vi "Main.vi"(11 "Module Admin":refnum<class "Delacor_lib_QMH_Cloneable Module Admin.lvclass">) -> ()   [LabVIEW 2025, in "Wheatstone Bridge.lvlib"]
doc: "This template is based off of the Queued Message Handler design pattern and the Queued Message Handler project template that ships with LabVIEW.\n\nThe main difference is that the queue is private to this module and communication between modules is performed via Broadcast and Request events.\n\nRequest events are wrapped in public API methods and are handled in the Event Handling Loop (EHL) of this VI. Any module can register for Broadcast events sent by this module. The EHL generates messages based on user interface actions.\n\nThe Message Handling Loop (MHL) processes messages generated by the EHL, or by other messages. The messages are string values, so new messages can be added easily to the Message Cases case structure in the MHL. Each message cluster can also provide an optional value for Message Data, which is a variant that can be converted to whatever message-specific data is required.\n_____\nBased on DQMH Dev Tools: Project Template 7.1.2.1547."
uses:
  Wheatstone Bridge.lvlib
  <vilib>/Delacor/Delacor QMH/Libraries/Message Queue_class/Delacor_lib_QMH_Message Queue.lvclass
  Module Data--cluster.ctl
  <vilib>/Utility/miscctls.llb/LVPointTypeDef.ctl
  <vilib>/Delacor/Delacor QMH/Libraries/Message Queue_class/Delacor_lib_QMH_Enqueue Message (Single).vi
  Stop Argument--cluster.ctl
  <vilib>/Delacor/Delacor QMH/Libraries/Cloneable Module Admin_class/Delacor_lib_QMH_Cloneable Module Admin.lvclass
  select child (Reply Payload)--cluster.ctl
  Wheatstone Bridge/Hardware Selection.ctl
  Wheatstone Bridge/Wheatstone Bridge.lvclass
  select child Argument--cluster.ctl
  NI-9237/NI-9237.lvclass
  read config (Reply Payload)--cluster.ctl
  read config Argument--cluster.ctl
  init device (Reply Payload)--cluster.ctl
  init device Argument--cluster.ctl
  close (Reply Payload)--cluster.ctl
  close Argument--cluster.ctl
  read data (Reply Payload)--cluster.ctl
  read data Argument--cluster.ctl
  read dvr (Reply Payload)--cluster.ctl
  read dvr Argument--cluster.ctl
  C:/Users/Tyson.Grover/Desktop/Repositories/torque-test-station/Libraries/Wheatstone Bridge/Wheatstone Bridge/Wheatstone Bridge.lvclass
  C:/Users/Tyson.Grover/Desktop/Repositories/torque-test-station/Libraries/Wheatstone Bridge/NI-9237/NI-9237.lvclass
panel:
  out "Stop the VI":bool
  out "Data Cluster":T1={"Status"="Inactive", "Wheatstone Bridge"=refnum}
  out "error out":errorcluster
  out "Status":string
  in  "Simulate EHL Error":bool
  in  "Simulate MHL Error":bool
  # "Other processes communicate with this Module via its Public API (wrappers for its Request Events).\n\nThis Module communicates with other processes via its Broadcast Events.\nAny process that wants to receive these messages can register for this module's Broadcast events."
  # "This template is for the DQMH framework. See the block diagram for more information on how to use this template."
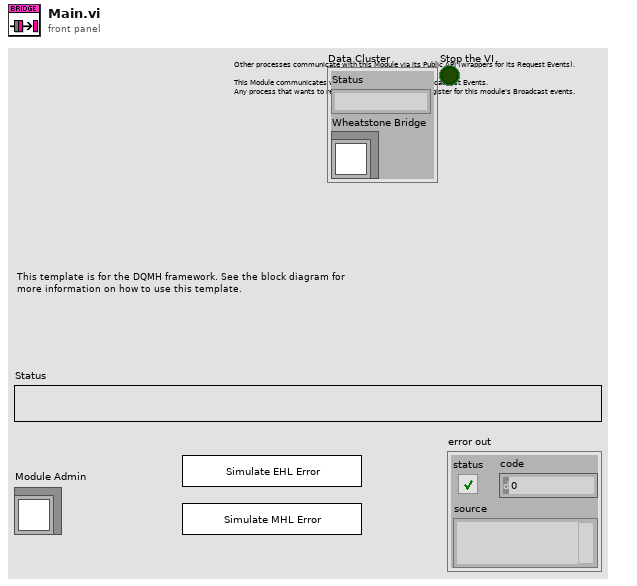
[diagram p1: front panel]
types:
  T1 = typedef "Wheatstone Bridge.lvlib/Module Data--cluster.ctl" = cluster{"Status":string, "Wheatstone Bridge":refnum<class "Wheatstone Bridge.lvclass">}
  T2 = typedef "Wheatstone Bridge.lvlib/Request Events--cluster.ctl" = cluster{"Stop Module":refnum<user-event>, "Show Panel":refnum<user-event>, "Hide Panel":refnum<user-event>, "Show Diagram":refnum<user-event>, "Get Module Execution Status":refnum<user-event>, "select child":refnum<user-event>, "read config":refnum<user-event>, "init":refnum<user-event>, "init device":refnum<user-event>, "close":refnum<user-event>, "read data":refnum<user-event>, "read dvr":refnum<user-event>}
  T3 = enum32{"invalid lock state", "Not Locked", "Locked (No Password)", "Password-protected"}
  T4 = typedef "Wheatstone Bridge.lvlib/Stop Argument--cluster.ctl" = cluster{"Module ID":i32, "Origin":string, "Exit via Stop Module Req?":bool, "Wait for Module to stop?":bool}
  T5 = typedef "Wheatstone Bridge.lvlib/select child Argument--cluster.ctl" = cluster{"Module ID":i32, "Hardware Selection":T6, "Wait Notifier":refnum<notifier>, "wait for reply":bool}
  T6 = typedef "Wheatstone Bridge.lvlib/Wheatstone Bridge.lvclass/Hardware Selection.ctl" = enum16{"Wheatstone Bridge", "NI-9237"}
  T7 = typedef "Wheatstone Bridge.lvlib/read config Argument--cluster.ctl" = cluster{"Module ID":i32, "File Path":path, "Wait Notifier":refnum<notifier>, "wait for reply":bool}
  T8 = typedef "Wheatstone Bridge.lvlib/init device Argument--cluster.ctl" = cluster{"Module ID":i32, "Variant":variant, "Wait Notifier":refnum<notifier>, "wait for reply":bool}
  T9 = typedef "Wheatstone Bridge.lvlib/close Argument--cluster.ctl" = cluster{"Module ID":i32, "Wait Notifier":refnum<notifier>, "wait for reply":bool}
  T10 = typedef "Wheatstone Bridge.lvlib/read data Argument--cluster.ctl" = cluster{"Module ID":i32, "Wait Notifier":refnum<notifier>, "wait for reply":bool}
  T11 = typedef "Wheatstone Bridge.lvlib/read dvr Argument--cluster.ctl" = cluster{"Module ID":i32, "Wait Notifier":refnum<notifier>, "wait for reply":bool}
  T12 = typedef "LVPointTypeDef.ctl" = cluster{"Horizontal":i16, "Vertical":i16}
  T13 = enum32{"Invalid", "Standard", "Closed", "Hidden", "Minimized", "Maximized"}
  T14 = typedef "Wheatstone Bridge.lvlib/select child (Reply Payload)--cluster.ctl" = cluster{"Module ID":i32, "error":errorcluster}
  T15 = typedef "Wheatstone Bridge.lvlib/read config (Reply Payload)--cluster.ctl" = cluster{"Module ID":i32, "error":errorcluster}
  T16 = typedef "Wheatstone Bridge.lvlib/init device (Reply Payload)--cluster.ctl" = cluster{"Module ID":i32, "error":errorcluster}
  T17 = typedef "Wheatstone Bridge.lvlib/close (Reply Payload)--cluster.ctl" = cluster{"Module ID":i32, "error":errorcluster}
  T18 = typedef "Wheatstone Bridge.lvlib/read data (Reply Payload)--cluster.ctl" = cluster{"Module ID":i32, "error":errorcluster}
  T19 = typedef "Wheatstone Bridge.lvlib/read dvr (Reply Payload)--cluster.ctl" = cluster{"Module ID":i32, "Numeric":dbl, "error":errorcluster}
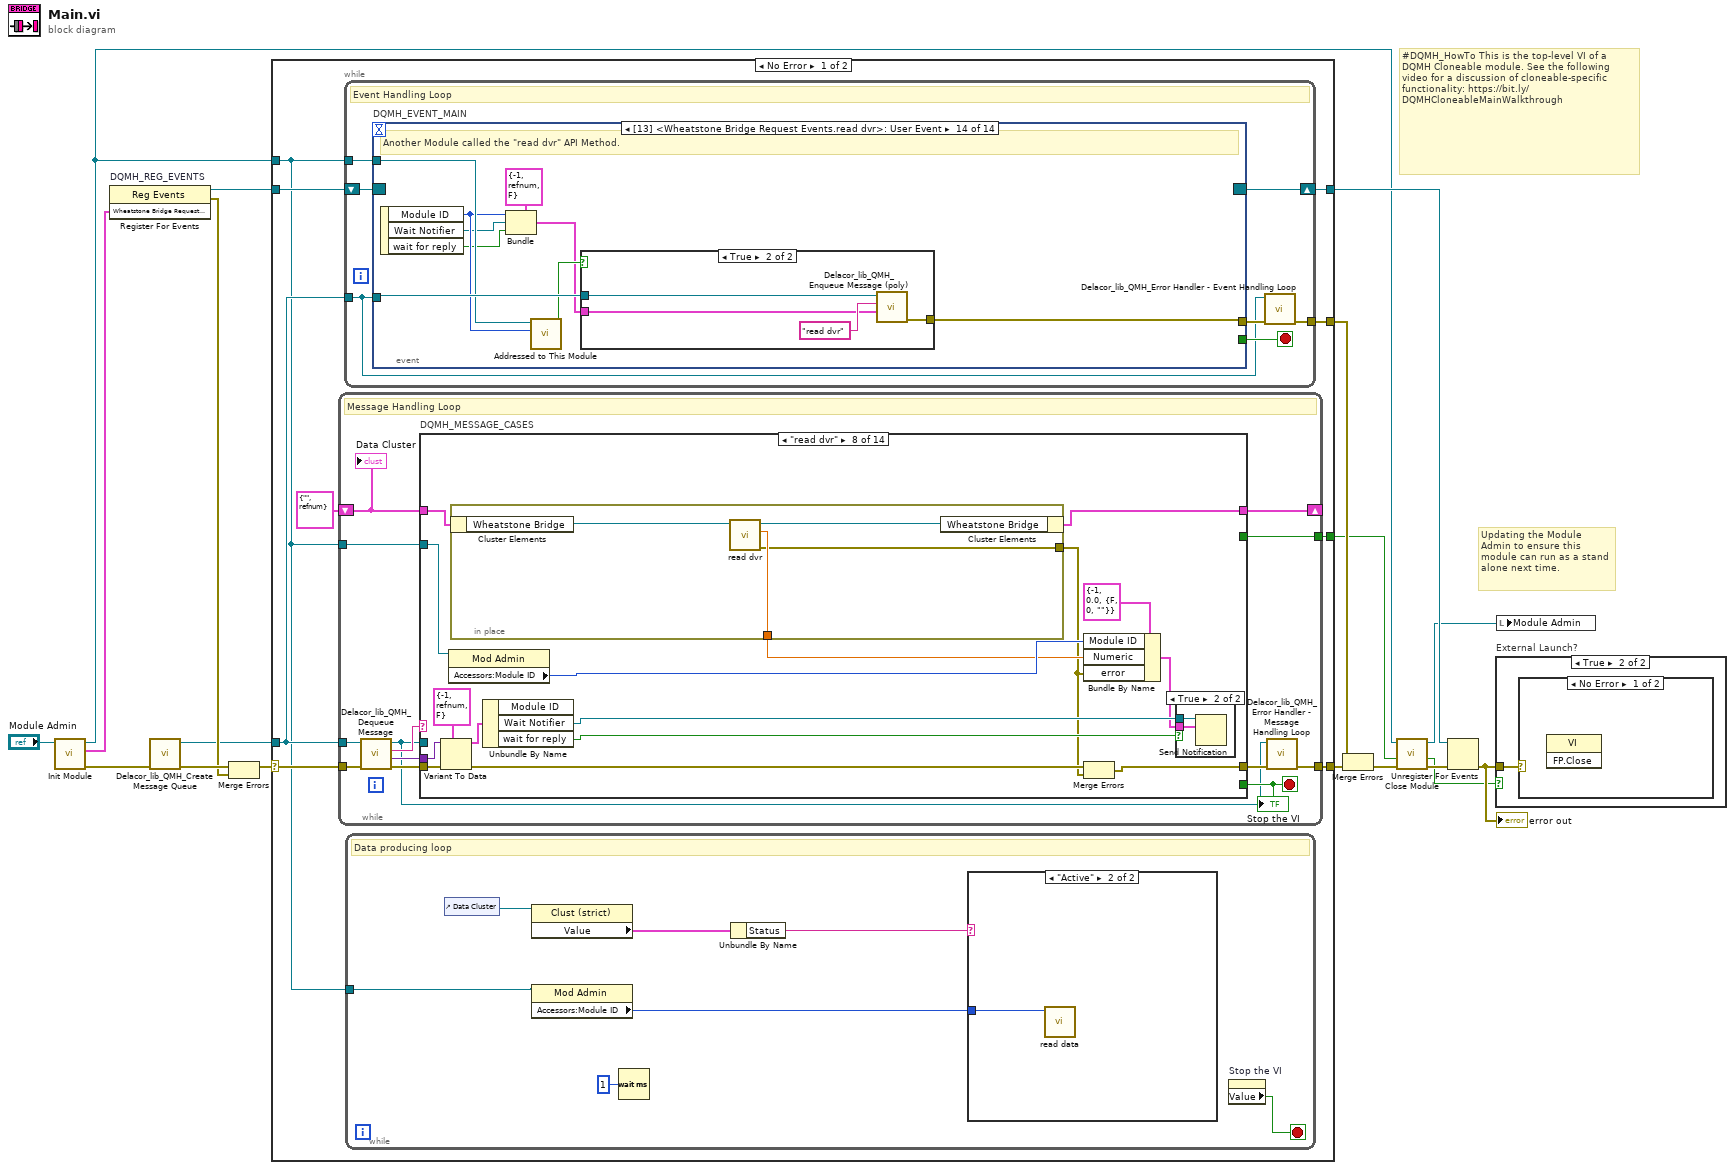
[diagram p0: block diagram]
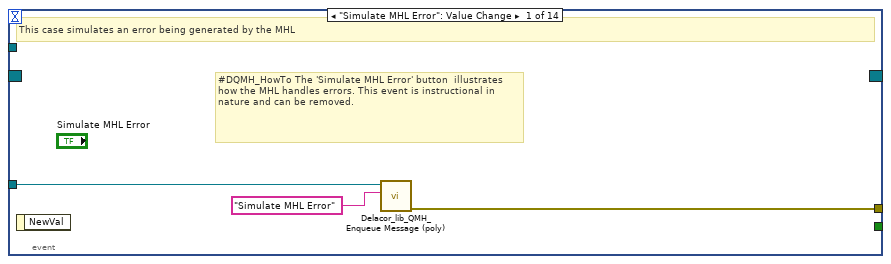
[diagram p3: hidden frame]
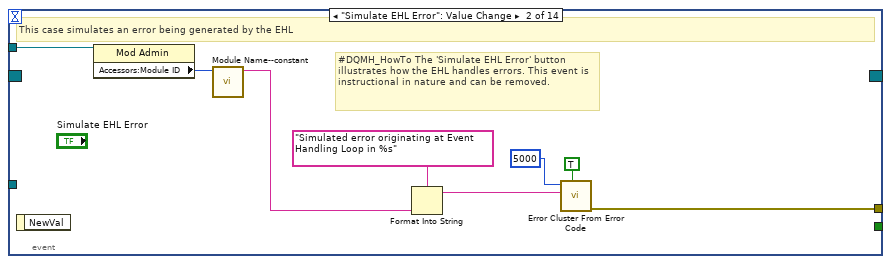
[diagram p4: hidden frame]
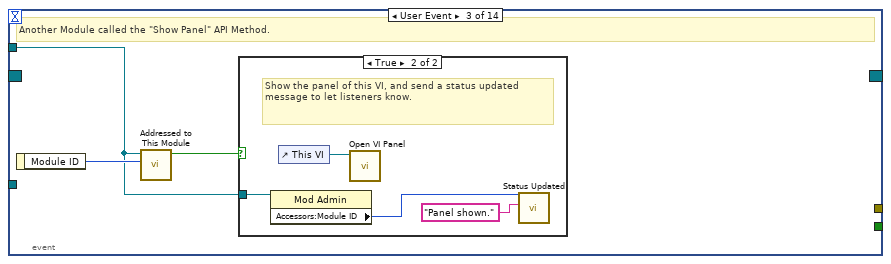
[diagram p5: hidden frame]
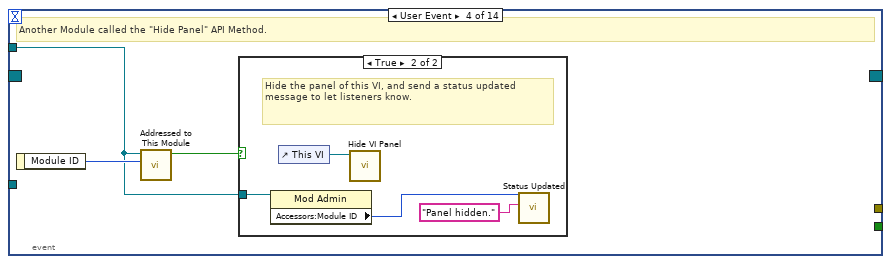
[diagram p7: hidden frame]
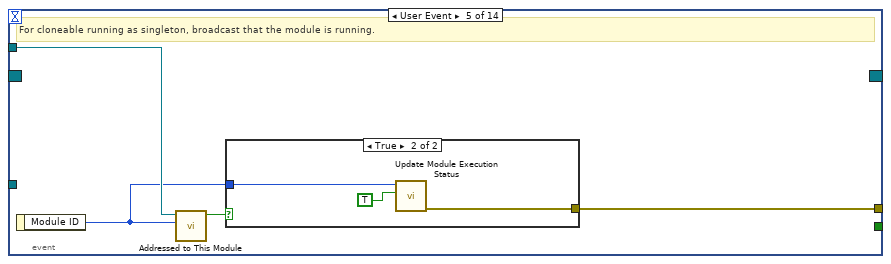
[diagram p9: hidden frame]
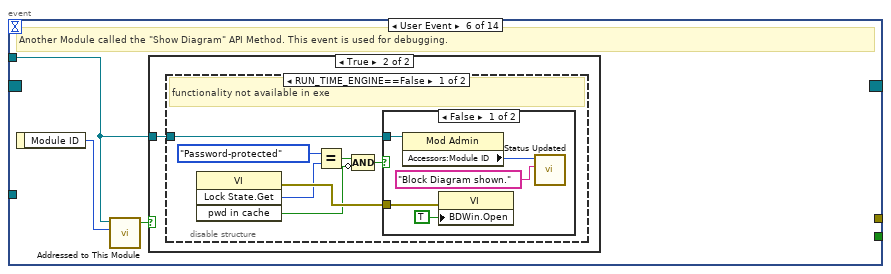
[diagram p11: hidden frame]
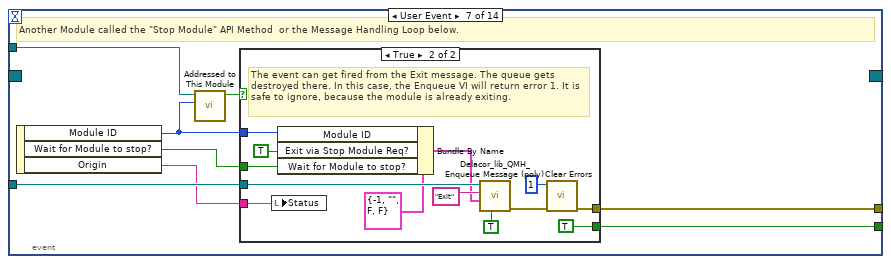
[diagram p15: hidden frame]
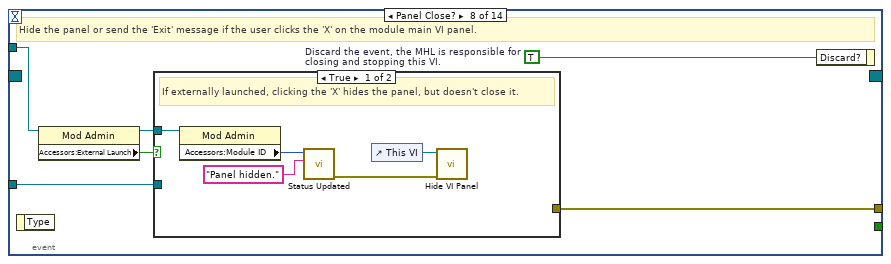
[diagram p17: hidden frame]
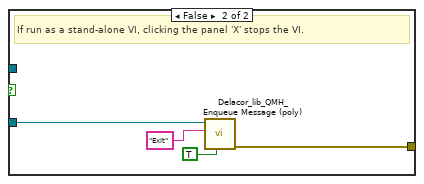
[diagram p18: hidden frame]
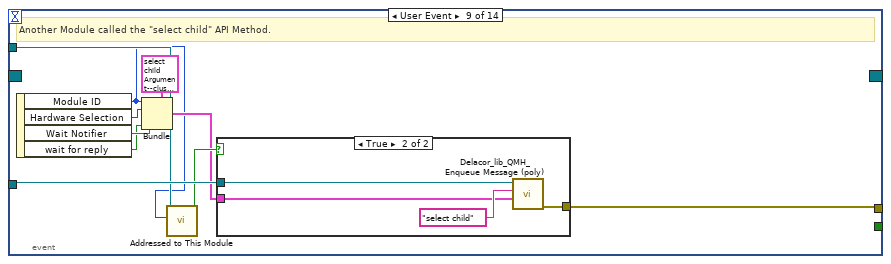
[diagram p19: hidden frame]
diagram:
  # "#DQMH_HowTo This is the top-level VI of a DQMH Cloneable module. See the following video for a discussion of cloneable-specific functionality: https://bit.ly/DQMHCloneableMainWalkthrough"
  # "Updating the Module Admin to ensure this module can run as a stand alone next time."
  n1 = call "Init Module.vi"("Cloneable Module Admin in"="Module Admin") -> ("error out"=w15:errorcluster, "Wheatstone Bridge Request Events"=w7:T2, "Cloneable Module Admin out"=w4:refnum<class "Delacor_lib_QMH_Cloneable Module Admin.lvclass">)  [unwired: 8 in]
  n2 = register-events "DQMH_REG_EVENTS"(w7) -> (reference out=w8:refnum<event-registration>, error out=w10:errorcluster)  [unwired: 2 in]
  n3 = call <vilib>:"Delacor_lib_QMH_Create Message Queue.vi"("error in"=w15) -> ("error out"=w12:errorcluster, "Message Queue"=w6:refnum<class "Delacor_lib_QMH_Message Queue.lvclass">)  [unwired: 9 in]
  n4 = Merge Errors(w12, w10) -> (w11:errorcluster)
  n5 = case shown="No Error" w11 {
    selector: w11 -> [w25 w448]
    tunnel: [w27 w447] -> w16
    tunnel: [w24 w446] -> w9
    tunnel: w8 -> [w22 w446]
    tunnel: w6 -> [w21 w439]
    tunnel: [w26 _] -> w17
    tunnel: w4 -> [w19 w442]
    tunnel: [w20 _] -> w2
    frame No Error {
      n6 = while {
        tunnel: w21 -> [w208]
        shift-right: [w215] -> _
        shift-left: T1 {"Status"="", "Wheatstone Bridge"=refnum} ("Data Cluster") -> [w216]
        tunnel: w25 -> [w219]
        tunnel: [w217] -> w27
        tunnel: w19 -> [w210]
        tunnel: [w209] -> w20
        stop <- w214 stop-if-true
        # "Message Handling Loop"
        n7 = call-dynamic "Delacor_lib_QMH_Dequeue Message.vi"("error in"=w219, "Message Queue in"=w208) -> ("error out"=w218:errorcluster, "Message Data"=w212:variant, "Message"=w213:string, "Message Queue out"=w211:refnum<class "Delacor_lib_QMH_Message Queue.lvclass">)  [unwired: 6 in]
        n8 = case "DQMH_MESSAGE_CASES" shown="\"read dvr\"" w213 {
          selector: w213 -> [_ _ _ _ _ _ _ _ _ _ _ _ _ w428]
          tunnel: w211 -> [_ _ _ _ _ _ _ _ _ _ w383 _ w420 _]
          tunnel: w218 -> [w239 w243 w259 w281 w303 w327 w348 w369 w378 w380 w392 w409 w426 w437]
          tunnel: [w237 w243 w250 w272 w294 w318 w339 w360 w377 w380 w388 w408 w421 w438] -> w220
          tunnel: w216 -> [w230 w242 w247 w269 w291 w315 w336 w357 w376 w379 w387 w406 w419 w435]
          tunnel: [w229 w242 w246 w268 w290 w314 w335 w356 w376 w379 w387 w406 w419 w435] -> w215
          tunnel: [_ _ _ _ _ _ _ _ _ _ _ _ w418 _] -> w214
          tunnel: w212 -> [_ _ w257 w279 w301 w325 w346 w367 _ _ w386 _ w416 _]
          tunnel: w210 -> [w225 _ w248 w270 w292 w316 w337 w358 _ _ w385 w404 w411 w434]
          tunnel: [_ _ _ _ _ _ _ _ _ _ _ _ w414 _] -> w209
          frame "Initialize" {
            w222 = "Initial Message" ("Initial Message")
            # "#DQMH_CodeNeeded - Initialize the appearance of the front panel."
            # "#DQMH_CodeNeeded - Initialize your state data here."
            # "Initialize - Any operation that needs to be done before the module can receive messages. Synchronize Caller Events.vi will inform Start Module.vi that the module has launched and is ready to receive messages. Module Did Init.vi will broadcast that the module initialized."
            n9 = call "Synchronize Caller Events.vi"("error in"=w239, "Module Admin"=w225) -> ("error out"=w238:errorcluster, "Module Admin out"=w224:refnum<class "Delacor_lib_QMH_Cloneable Module Admin.lvclass">)  [unwired: 8 in]
            n10 = property on="Property Node" class="Mod Admin"(reference=w224) -> ("Accessors:Module ID"=w221:i32, "Accessors:External Launch"=w226:bool)  [unwired: 1 in, 2 out]
            n11 = call "Module Name--constant.vi"("Module ID"=w221) -> ("Module Name"=w234:string)  [unwired: 10 in]
            n12 = property on="Property Node" class="VI"("Front Panel.Title"=w234) -> (reference out=w236:refnum<vi>, error out=w241:errorcluster)  [unwired: 2 in]
            n13 = Select(t=T13."Hidden" ("State"), s=w226, f=T13."Standard" ("State")) -> (s? t:f=w231:T13)
            n14 = invoke on="Invoke Node" class="VI" method="FP.Open"(reference=w236, error in=w241, "State"=w231) -> (reference out=w235:refnum<vi>, error out=w240:errorcluster)  [unwired: 2 in, 3 out]
            n15 = Bundle By Name(cluster=w230, "Status"=w222) -> (w229:T1)
            n16 = invoke on="Invoke Node" class="VI" method="FP.Center"(reference=w235, error in=w240) -> ()  [unwired: 1 in, 3 out]
            n17 = property on="Pane" class="Pane"("Origin"=T12 {"Horizontal"=0, "Vertical"=0}) -> ()  [unwired: 2 in, 2 out]
            n18 = call "Module Name--constant.vi"("Module ID"=w221) -> ("Module Name"=w227:string)  [unwired: 10 in]
            n19 = call "Module Did Init.vi"("error in"=w238, "Initialized?"=TRUE, "Origin"=w227, "Module ID"=w221) -> ("error out"=w237:errorcluster)  [unwired: 7 in]
            "Status" <- w222
          }
          frame "---Module Specific---" {
            # "Separator -- The following cases handle messages specific to this Module."
          }
          frame "select child" {
            w244 = errorcluster {"status"=FALSE, "code"=0, "source"=""} ("error")
            n20 = property class="Mod Admin"(reference=w248) -> ("Accessors:Module ID"=w249:i32)  [unwired: 1 in, 2 out]
            n21 = Variant To Data(error in=w259, type=T5 {"Module ID"=-1, "Hardware Selection"=enum."Wheatstone Bridge", "Wait Notifier"=refnum, "wait for reply"=FALSE} ("select child Argument"), Variant=w257) -> (data=w255:T5, error out=w258:errorcluster)
            n22 = Unbundle By Name(w255) -> ("Hardware Selection"=w245:T6, "Wait Notifier"=w254:refnum<notifier>, "wait for reply"=w253:bool)  [unwired: 1 out]
            n23 = in-place {
              in-place-border: w245 -> [w261]
              n24 = in-place-cluster #1(w247) -> ()  [unwired: 1 out]
              n25 = case shown="\"Wheatstone Bridge\", Default" w261 {
                tunnel: [refnum<class "Wheatstone Bridge.lvclass"> refnum ("Wheatstone Bridge.lvlib:Wheatstone Bridge.lvclass") refnum<class "NI-9237.lvclass"> refnum ("Wheatstone Bridge.lvlib:NI-9237.lvclass")] -> w260
                frame "Wheatstone Bridge", Default {
                }
                frame "NI-9237" {
                }
              }
              n26 = in-place-cluster #1("Wheatstone Bridge"=w260) -> (w246:T1)
            }
            n27 = Bundle By Name(cluster=T14 {"Module ID"=-1, "error"={"status"=FALSE, "code"=0, "source"=""}} ("select child (Reply Payload)"), "Module ID"=w249, "error"=w244) -> (w252:T14)
            n28 = Merge Errors(w258, w244) -> (w250:errorcluster)
            n29 = case "DQMH_FIRE_NOTIFIER" shown="True" w253 {
              tunnel: w254 -> [_ w265]
              tunnel: w252 -> [_ w264]
              frame False {
              }
              frame True {
                n30 = Send Notification(notification=w264, notifier=w265) -> ()  [unwired: 1 in, 2 out]
              }
            }
          }
          frame "read config" {
            n31 = property class="Mod Admin"(reference=w270) -> ("Accessors:Module ID"=w271:i32)  [unwired: 1 in, 2 out]
            n32 = Variant To Data(error in=w281, type=T7 {"Module ID"=-1, "File Path"=path "", "Wait Notifier"=refnum, "wait for reply"=FALSE} ("read config Argument"), Variant=w279) -> (data=w277:T7, error out=w280:errorcluster)
            n33 = Unbundle By Name(w277) -> ("File Path"=w266:path, "Wait Notifier"=w276:refnum<notifier>, "wait for reply"=w275:bool)  [unwired: 1 out]
            n34 = in-place {
              in-place-border: [w284] -> w267
              in-place-border: w266 -> [w282]
              n35 = in-place-cluster #2(w269) -> ("Wheatstone Bridge"=w283:refnum<class "Wheatstone Bridge.lvclass">)
              n36 = call-dynamic "read config.vi"("File Path"=w282, "Wheatstone Bridge in"=w283) -> ("error out"=w284:errorcluster, "Wheatstone Bridge out"=w285:refnum<class "Wheatstone Bridge.lvclass">)  [unwired: 8 in]
              n37 = in-place-cluster #2("Wheatstone Bridge"=w285) -> (w268:T1)
            }
            n38 = Bundle By Name(cluster=T15 {"Module ID"=-1, "error"={"status"=FALSE, "code"=0, "source"=""}} ("read config (Reply Payload)"), "Module ID"=w271, "error"=w267) -> (w274:T15)
            n39 = Merge Errors(w280, w267) -> (w272:errorcluster)
            n40 = case "DQMH_FIRE_NOTIFIER" shown="True" w275 {
              tunnel: w276 -> [_ w287]
              tunnel: w274 -> [_ w286]
              frame False {
              }
              frame True {
                n41 = Send Notification(notification=w286, notifier=w287) -> ()  [unwired: 1 in, 2 out]
              }
            }
          }
          frame "init device" {
            n42 = property class="Mod Admin"(reference=w292) -> ("Accessors:Module ID"=w293:i32)  [unwired: 1 in, 2 out]
            n43 = Variant To Data(error in=w303, type=T8 {"Module ID"=-1, "Variant"=variant, "Wait Notifier"=refnum, "wait for reply"=FALSE} ("init device Argument"), Variant=w301) -> (data=w299:T8, error out=w302:errorcluster)
            n44 = Unbundle By Name(w299) -> ("Variant"=w288:variant, "Wait Notifier"=w298:refnum<notifier>, "wait for reply"=w297:bool)  [unwired: 1 out]
            n45 = in-place {
              in-place-border: [w305] -> w289
              in-place-border: w288 -> [w306]
              n46 = in-place-cluster #3(w291) -> ("Wheatstone Bridge"=w307:refnum<class "Wheatstone Bridge.lvclass">)  [unwired: 1 out]
              n47 = call-dynamic "init.vi"("Variant"=w306, "Wheatstone Bridge in"=w307) -> ("error out"=w305:errorcluster, "Wheatstone Bridge out"=w308:refnum<class "Wheatstone Bridge.lvclass">)  [unwired: 8 in]
              n48 = case shown="No Error" w305 {
                tunnel: ["Active" ("Status") "Error" ("Status")] -> w304
                frame No Error {
                }
                frame Error {
                }
              }
              n49 = in-place-cluster #3("Wheatstone Bridge"=w308, "Status"=w304) -> (w290:T1)
            }
            n50 = Bundle By Name(cluster=T16 {"Module ID"=-1, "error"={"status"=FALSE, "code"=0, "source"=""}} ("init device (Reply Payload)"), "Module ID"=w293, "error"=w289) -> (w296:T16)
            n51 = Merge Errors(w302, w289) -> (w294:errorcluster)
            n52 = case "DQMH_FIRE_NOTIFIER" shown="True" w297 {
              tunnel: w298 -> [_ w312]
              tunnel: w296 -> [_ w311]
              frame False {
              }
              frame True {
                n53 = Send Notification(notification=w311, notifier=w312) -> ()  [unwired: 1 in, 2 out]
              }
            }
          }
          frame "close" {
            n54 = Variant To Data(error in=w327, type=T9 {"Module ID"=-1, "Wait Notifier"=refnum, "wait for reply"=FALSE} ("close Argument"), Variant=w325) -> (data=w323:T9, error out=w326:errorcluster)
            n55 = property class="Mod Admin"(reference=w316) -> ("Accessors:Module ID"=w317:i32)  [unwired: 1 in, 2 out]
            n56 = in-place {
              in-place-border: [w329] -> w313
              n57 = in-place-cluster #4(w315) -> ("Wheatstone Bridge"=w330:refnum<class "Wheatstone Bridge.lvclass">)  [unwired: 1 out]
              n58 = call-dynamic "close.vi"("Wheatstone Bridge in"=w330) -> ("error out"=w329:errorcluster, "Wheatstone Bridge out"=w331:refnum<class "Wheatstone Bridge.lvclass">)  [unwired: 9 in]
              n59 = in-place-cluster #4("Wheatstone Bridge"=w331, "Status"="Inactive") -> (w314:T1)
            }
            n60 = Unbundle By Name(w323) -> ("Wait Notifier"=w322:refnum<notifier>, "wait for reply"=w321:bool)  [unwired: 1 out]
            n61 = Bundle By Name(cluster=T17 {"Module ID"=-1, "error"={"status"=FALSE, "code"=0, "source"=""}} ("close (Reply Payload)"), "Module ID"=w317, "error"=w313) -> (w320:T17)
            n62 = Merge Errors(w326, w313) -> (w318:errorcluster)
            n63 = case "DQMH_FIRE_NOTIFIER" shown="True" w321 {
              tunnel: w322 -> [_ w333]
              tunnel: w320 -> [_ w332]
              frame False {
              }
              frame True {
                n64 = Send Notification(notification=w332, notifier=w333) -> ()  [unwired: 1 in, 2 out]
              }
            }
          }
          frame "read data" {
            n65 = property class="Mod Admin"(reference=w337) -> ("Accessors:Module ID"=w338:i32)  [unwired: 1 in, 2 out]
            n66 = Variant To Data(error in=w348, type=T10 {"Module ID"=-1, "Wait Notifier"=refnum, "wait for reply"=FALSE} ("read data Argument"), Variant=w346) -> (data=w344:T10, error out=w347:errorcluster)
            n67 = in-place {
              in-place-border: [w349] -> w334
              n68 = in-place-cluster #5(w336) -> ("Wheatstone Bridge"=w351:refnum<class "Wheatstone Bridge.lvclass">)
              n69 = call-dynamic "read data.vi"("Wheatstone Bridge in"=w351) -> ("error out"=w349:errorcluster, "Wheatstone Bridge out"=w350:refnum<class "Wheatstone Bridge.lvclass">)  [unwired: 9 in]
              n70 = in-place-cluster #5("Wheatstone Bridge"=w350) -> (w335:T1)
            }
            n71 = Unbundle By Name(w344) -> ("Wait Notifier"=w343:refnum<notifier>, "wait for reply"=w342:bool)  [unwired: 1 out]
            n72 = Bundle By Name(cluster=T18 {"Module ID"=-1, "error"={"status"=FALSE, "code"=0, "source"=""}} ("read data (Reply Payload)"), "Module ID"=w338, "error"=w334) -> (w341:T18)
            n73 = Merge Errors(w347, w334) -> (w339:errorcluster)
            n74 = case "DQMH_FIRE_NOTIFIER" shown="True" w342 {
              tunnel: w343 -> [_ w353]
              tunnel: w341 -> [_ w352]
              frame False {
              }
              frame True {
                n75 = Send Notification(notification=w352, notifier=w353) -> ()  [unwired: 1 in, 2 out]
              }
            }
          }
          frame "read dvr" {
            n76 = Variant To Data(error in=w369, type=T11 {"Module ID"=-1, "Wait Notifier"=refnum, "wait for reply"=FALSE} ("read dvr Argument"), Variant=w367) -> (data=w365:T11, error out=w368:errorcluster)
            n77 = property class="Mod Admin"(reference=w358) -> ("Accessors:Module ID"=w359:i32)  [unwired: 1 in, 2 out]
            n78 = in-place {
              in-place-border: [w371] -> w355
              in-place-border: [w370] -> w354
              n79 = in-place-cluster #6(w357) -> ("Wheatstone Bridge"=w372:refnum<class "Wheatstone Bridge.lvclass">)
              n80 = call-dynamic "read dvr.vi"("Wheatstone Bridge in"=w372) -> ("error out"=w370:errorcluster, "Numeric"=w371:dbl, "Wheatstone Bridge out"=w373:refnum<class "Wheatstone Bridge.lvclass">)  [unwired: 8 in]
              n81 = in-place-cluster #6("Wheatstone Bridge"=w373) -> (w356:T1)
            }
            n82 = Unbundle By Name(w365) -> ("Wait Notifier"=w364:refnum<notifier>, "wait for reply"=w363:bool)  [unwired: 1 out]
            n83 = Bundle By Name(cluster=T19 {"Module ID"=-1, "Numeric"=0.0, "error"={"status"=FALSE, "code"=0, "source"=""}} ("read dvr (Reply Payload)"), "Module ID"=w359, "Numeric"=w355, "error"=w354) -> (w362:T19)
            n84 = Merge Errors(w368, w354) -> (w360:errorcluster)
            n85 = case "DQMH_FIRE_NOTIFIER" shown="True" w363 {
              tunnel: w364 -> [_ w375]
              tunnel: w362 -> [_ w374]
              frame False {
              }
              frame True {
                n86 = Send Notification(notification=w374, notifier=w375) -> ()  [unwired: 1 in, 2 out]
              }
            }
          }
          frame "---Copy This Frame---" {
            # "Duplicate this frame when creating new messages.  Change this comment in the duplicated frame to describe this message."
            n87 = Merge Errors(w378) -> (w377:errorcluster)
          }
          frame "---Exit and Error Handling---" {
            # "Separator - the following cases handle errors and exit messages."
          }
          frame "Error" {
            # "#DQMH_CodeRecommended - If the module is running in standalone mode (External Launch = FALSE), this code will pop up an error dialog and call the 'Exit' message if an error occurs. Add more fine-grained error management here."
            # "Error - Check the error message data and respond accordingly. This message is sent by the \"Error Handler\" VIs at the end of each loop in this application."
            n88 = property on="Property Node" class="Mod Admin"(reference=w385) -> ("Accessors:External Launch"=w384:bool, "Accessors:Module ID"=w382:i32)  [unwired: 1 in, 2 out]
            n89 = Variant To Data(error in=w392, type=errorcluster {"status"=FALSE, "code"=0, "source"=""} ("error constant"), Variant=w386) -> (data=w381:errorcluster, error out=w390:errorcluster)
            n90 = local write "error out"(w381) -> ()
            n91 = call "Error Reported.vi"("Error"=w381, "Module ID"=w382) -> ()  [unwired: 9 in, 1 out]
            n92 = case shown="False" w384 {
              tunnel: [w397 _] -> w389
              tunnel: w383 -> [w395 _]
              tunnel: w381 -> [w396 _]
              frame False {
                n93 = disable-structure shown="Default" {
                  disable-tunnel: w396 -> [w398 _]
                  frame condition #0 (active) {
                    # "If the module is running standalone, then pop up an error dialog and call the \"Exit\" message."
                    n94 = call <vilib>:"Simple Error Handler.vi"("error in (no error)"=w398) -> ()  [unwired: 4 in, 5 out]
                  }
                  frame condition #1 {
                    # "To prevent the Simple Error Handler VI from being loaded (e.g. when deploying to a Real-Time target), add the Conditional Disable Symbol \"DQMH_Disable_SEH\" to your project and set it to TRUE."
                  }
                }
                n95 = call-poly <vilib>:"Delacor_lib_QMH_Enqueue Message (poly).vi"("Priority Message? (F)"=TRUE, "Message"="Exit", "Message Queue in"=w395) -> ("error out"=w397:errorcluster)  [unwired: 7 in, 1 out]
              }
              frame True {
                # "If the module was launched externally, calling the Error Reported broadcast VI is the only action performed by the \"Error\" message. The module's caller can then process the error appropriately."
              }
            }
            n96 = Merge Errors(w390, w389) -> (w388:errorcluster)
          }
          frame "Simulate MHL Error" {
            # "#DQMH_HowTo The 'Simulate MHL Error' button  illustrates how the MHL handles errors. This event is instructional in nature and can be removed."
            # "Simulate an error occurring at the MHL"
            n97 = property on="Property Node" class="Mod Admin"(reference=w404) -> ("Accessors:Module ID"=w405:i32)  [unwired: 1 in, 2 out]
            n98 = call "Module Name--constant.vi"("Module ID"=w405) -> ("Module Name"=w400:string)  [unwired: 10 in]
            n99 = Format Into String(format string="Simulated error originating at Message Handling Loop in %s", w400) -> (resulting string=w401:string)  [unwired: 2 in, 1 out]
            n100 = call <vilib>:"Error Cluster From Error Code.vi"("show call chain? (False)"=TRUE, "error message (\"\")"=w401, "error code (0)"=5001) -> ("error out"=w407:errorcluster)  [unwired: 6 in]
            n101 = Merge Errors(w409, w407) -> (w408:errorcluster)
          }
          frame "Exit" {
            w417 = 91  # 91: not all Exit messages will have an argument
            w418 = TRUE  # Stop the VI
            # "Release the message queue reference"
            # "#DQMH_CodeNeeded - Add any required cleanup code here."
            # "Exit - Exit the application."
            n102 = Variant To Data(error in=w426, type=T4 {"Module ID"=-1, "Origin"="", "Exit via Stop Module Req?"=FALSE, "Wait for Module to stop?"=FALSE} ("Stop Argument"), Variant=w416) -> (data=w413:T4, error out=w422:errorcluster)
            n103 = call <vilib>:"Clear Errors.vi"("error in (no error)"=w422, "specific error code to clear (0: all)"=w417) -> ("error out"=w425:errorcluster)  [unwired: 4 in, 1 out]
            n104 = property on="Property Node" class="Mod Admin"(reference=w411) -> ("Accessors:Module ID"=w410:i32)  [unwired: 1 in, 2 out]
            n105 = control-ref of="This VI"() -> (w412:refnum<vi>)
            n106 = call-dynamic "Delacor_lib_QMH_Release Message Queue.vi"("error in"=w425, "Message Queue"=w420) -> ("error out"=w424:errorcluster)  [unwired: 9 in]
            n107 = call "Handle Exit.vi"("Stop Argument"=w413, "Module Admin in"=w411, "VI reference"=w412) -> ("error out"=w423:errorcluster, "Wait for Stop?"=w414:bool)  [unwired: 7 in]
            n108 = Merge Errors(w424, w423) -> (w421:errorcluster)
            n109 = call "Error Reported.vi"("Error"=w421, "Module ID"=w410) -> ()  [unwired: 9 in, 1 out]
          }
          frame Default {
            # "'Default' case only runs if there is a message that isn't defined in any of the other cases.  Output a programming error."
            n110 = property on="Property Node" class="Mod Admin"(reference=w434) -> ("Accessors:Module ID"=w433:i32)  [unwired: 1 in, 2 out]
            n111 = call "Module Name--constant.vi"("Module ID"=w433) -> ("Module Name"=w427:string)  [unwired: 10 in]
            n112 = Format Into String(format string="The invalid message string \"%s\" was received in the Message Handling Loop for module \"%s\".", w428, w427) -> (resulting string=w430:string)  [unwired: 2 in, 1 out]
            n113 = call <vilib>:"Error Cluster From Error Code.vi"("show call chain? (False)"=TRUE, "error message (\"\")"=w430, "error code (0)"=1) -> ("error out"=w436:errorcluster)  [unwired: 6 in]
            n114 = Merge Errors(w437, w436) -> (w438:errorcluster)
          }
        }
        "Stop the VI" <- w214
        n115 = call-dynamic "Delacor_lib_QMH_Error Handler - Message Handling Loop.vi"("error in"=w220, "Message Queue in"=w211) -> ("dup error in"=w217:errorcluster)  [unwired: 8 in, 1 out]
        "Data Cluster" <- w216
      }
      n116 = while {
        tunnel: w21 -> [w36]
        shift-right: [w39] -> w24
        shift-left: w22 -> [w40]
        tunnel: [w41] -> w26
        tunnel: w19 -> [w37]
        stop <- w38 stop-if-true
        # "Event Handling Loop"
        n117 = event "DQMH_EVENT_MAIN" shown="[13] <Wheatstone Bridge Request Events.read dvr>: User Event" {
          selector: w40 -> [_ _ _ _ _ _ _ _ _ _ _ _ _ _]
          dyn-events: [_ _ _ _ _ _ _ _ _ _ _ _ _ _] -> w39
          timeout: _ -> [_ _ _ _ _ _ _ _ _ _ _ _ _ _]
          tunnel: [_ _ _ _ _ _ w94 _ _ _ _ _ _ _] -> w38
          tunnel: w36 -> [w44 _ _ _ _ _ w97 w114 w136 w150 w164 w177 w190 w203]
          tunnel: [w45 w53 _ _ w71 _ w98 w117 w127 w141 w155 w169 w182 w195] -> w42
          tunnel: w37 -> [_ w52 w54 w61 w69 w75 w96 w115 w134 w148 w162 w175 w188 w201]
          event "Simulate MHL Error": Value Change {
            # "#DQMH_HowTo The 'Simulate MHL Error' button  illustrates how the MHL handles errors. This event is instructional in nature and can be removed."
            # "This case simulates an error being generated by the MHL"
            n118 = event-data() -> ()  [unwired: 1 in, 1 out]
            n119 = call-poly <vilib>:"Delacor_lib_QMH_Enqueue Message (poly).vi"("Message"="Simulate MHL Error", "Message Queue in"=w44) -> ("error out"=w45:errorcluster)  [unwired: 8 in, 1 out]
          }
          event "Simulate EHL Error": Value Change {
            # "#DQMH_HowTo The 'Simulate EHL Error' button  illustrates how the EHL handles errors. This event is instructional in nature and can be removed."
            # "This case simulates an error being generated by the EHL"
            n120 = event-data() -> ()  [unwired: 1 in, 1 out]
            n121 = property on="Property Node" class="Mod Admin"(reference=w52) -> ("Accessors:Module ID"=w51:i32)  [unwired: 1 in, 2 out]
            n122 = call "Module Name--constant.vi"("Module ID"=w51) -> ("Module Name"=w46:string)  [unwired: 10 in]
            n123 = Format Into String(format string="Simulated error originating at Event Handling Loop in %s", w46) -> (resulting string=w49:string)  [unwired: 2 in, 1 out]
            n124 = call <vilib>:"Error Cluster From Error Code.vi"("show call chain? (False)"=TRUE, "error message (\"\")"=w49, "error code (0)"=5000) -> ("error out"=w53:errorcluster)  [unwired: 6 in]
          }
          event User Event {
            # "Another Module called the \"Show Panel\" API Method."
            n125 = event-data() -> ("Module ID"=w55:i32)  [unwired: 1 in]
            n126 = call "Addressed to This Module.vi"("Module ID from Argument"=w55, "Module Admin"=w54) -> ("Addressed to this instance?"=w56:bool)  [unwired: 8 in, 1 out]
            n127 = case shown="True" w56 {
              tunnel: w54 -> [_ w58]
              frame False {
              }
              frame True {
                # "Show the panel of this VI, and send a status updated message to let listeners know."
                n128 = property on="Property Node" class="Mod Admin"(reference=w58) -> ("Accessors:Module ID"=w57:i32)  [unwired: 1 in, 2 out]
                n129 = control-ref of="This VI"() -> (w60:refnum<vi>)
                n130 = call "Open VI Panel.vi"("VI"=w60) -> ()  [unwired: 10 in, 1 out]
                n131 = call "Status Updated.vi"("Status"="Panel shown." ("format string"), "Module ID"=w57) -> ()  [unwired: 9 in, 1 out]
              }
            }
          }
          event User Event {
            # "Another Module called the \"Hide Panel\" API Method."
            n132 = event-data() -> ("Module ID"=w62:i32)  [unwired: 1 in]
            n133 = call "Addressed to This Module.vi"("Module ID from Argument"=w62, "Module Admin"=w61) -> ("Addressed to this instance?"=w63:bool)  [unwired: 8 in, 1 out]
            n134 = case shown="True" w63 {
              tunnel: w61 -> [_ w65]
              frame False {
              }
              frame True {
                # "Hide the panel of this VI, and send a status updated message to let listeners know."
                n135 = property on="Property Node" class="Mod Admin"(reference=w65) -> ("Accessors:Module ID"=w64:i32)  [unwired: 1 in, 2 out]
                n136 = control-ref of="This VI"() -> (w67:refnum<vi>)
                n137 = call "Hide VI Panel.vi"("VI"=w67) -> ()  [unwired: 10 in, 1 out]
                n138 = call "Status Updated.vi"("Status"="Panel hidden." ("format string"), "Module ID"=w64) -> ()  [unwired: 9 in, 1 out]
              }
            }
          }
          event User Event {
            # "For cloneable running as singleton, broadcast that the module is running."
            n139 = event-data() -> ("Module ID"=w68:i32)  [unwired: 1 in]
            n140 = call "Addressed to This Module.vi"("Module ID from Argument"=w68, "Module Admin"=w69) -> ("Addressed to this instance?"=w70:bool)  [unwired: 8 in, 1 out]
            n141 = case shown="True" w70 {
              tunnel: [_ w74] -> w71
              tunnel: w68 -> [_ w73]
              frame False {
              }
              frame True {
                n142 = call "Update Module Execution Status.vi"("Running?"=TRUE, "Module ID"=w73) -> ("error out"=w74:errorcluster)  [unwired: 9 in]
              }
            }
          }
          event User Event {
            # "Another Module called the \"Show Diagram\" API Method. This event is used for debugging."
            n143 = event-data() -> ("Module ID"=w76:i32)  [unwired: 1 in]
            n144 = call "Addressed to This Module.vi"("Module ID from Argument"=w76, "Module Admin"=w75) -> ("Addressed to this instance?"=w77:bool)  [unwired: 8 in, 1 out]
            n145 = case shown="True" w77 {
              tunnel: w75 -> [_ w78]
              frame False {
              }
              frame True {
                n146 = disable-structure shown="RUN_TIME_ENGINE==False" {
                  disable-tunnel: w78 -> [w79 _]
                  frame condition #0 (active) {
                    # "functionality not available in exe"
                    n147 = invoke on="Invoke Node" class="VI" method="Lock State.Get"() -> (error out=w85:errorcluster, "Get Lock State"=w84:T3, "pwd in cache"=w81:bool)  [unwired: 4 in, 1 out]
                    n148 = Equal?(x=T3."Password-protected", y=w84) -> (x = y?=w82:bool)
                    n149 = Compound Arithmetic op=AND(w82, invert w81) -> (w80:bool)
                    n150 = case shown="False" w80 {
                      tunnel: w85 -> [w90 _]
                      tunnel: w79 -> [w87 _]
                      frame False {
                        n151 = property on="Property Node" class="Mod Admin"(reference=w87) -> ("Accessors:Module ID"=w86:i32)  [unwired: 1 in, 2 out]
                        n152 = property on="Property Node" class="VI"(error in=w90, "BDWin.Open"=TRUE ("Block Diagram Window:Open")) -> ()  [unwired: 1 in, 2 out]
                        n153 = call "Status Updated.vi"("Status"="Block Diagram shown." ("format string"), "Module ID"=w86) -> ()  [unwired: 9 in, 1 out]
                      }
                      frame True {
                        # "Password-protected VI, and the password is not in the cache. Do not show the diagram."
                      }
                    }
                  }
                  frame condition #1 {
                  }
                }
              }
            }
          }
          event User Event {
            # "Another Module called the \"Stop Module\" API Method  or the Message Handling Loop below."
            n154 = event-data() -> ("Module ID"=w92:i32, "Wait for Module to stop?"=w93:bool, "Origin"=w91:string)  [unwired: 1 in]
            n155 = call "Addressed to This Module.vi"("Module ID from Argument"=w92, "Module Admin"=w96) -> ("Addressed to this instance?"=w95:bool)  [unwired: 8 in, 1 out]
            n156 = case shown="True" w95 {
              tunnel: [_ w110] -> w98
              tunnel: w97 -> [_ w106]
              tunnel: [_ TRUE] -> w94
              tunnel: w93 -> [_ w101]
              tunnel: w92 -> [_ w103]
              tunnel: w91 -> [_ w99]
              frame False {
              }
              frame True {
                # "The event can get fired from the Exit message. The queue gets destroyed there. In this case, the Enqueue VI will return error 1. It is safe to ignore, because the module is already exiting."
                n157 = local write "Status"(w99) -> ()
                n158 = Bundle By Name(cluster=T4 {"Module ID"=-1, "Origin"="", "Exit via Stop Module Req?"=FALSE, "Wait for Module to stop?"=FALSE} ("Stop Argument"), "Module ID"=w103, "Exit via Stop Module Req?"=TRUE, "Wait for Module to stop?"=w101) -> (w100:T4)
                n159 = call-poly <vilib>:"Delacor_lib_QMH_Enqueue Message (poly).vi"("Priority Message? (F)"=TRUE, "Message Data"=w100, "Message"="Exit", "Message Queue in"=w106) -> ("error out"=w111:errorcluster)  [unwired: 6 in, 1 out]
                n160 = call <vilib>:"Clear Errors.vi"("error in (no error)"=w111, "specific error code to clear (0: all)"=1) -> ("error out"=w110:errorcluster)  [unwired: 4 in, 1 out]
              }
            }
          }
          event Panel Close? {
            w116 = TRUE  # Discard the event, the MHL is responsible for closing and stopping this VI.
            # "Hide the panel or send the 'Exit' message if the user clicks the 'X' on the module main VI panel."
            n161 = event-data() -> ()  [unwired: 1 in, 1 out]
            n162 = property on="Property Node" class="Mod Admin"(reference=w115) -> (reference out=w112:refnum<class "Delacor_lib_QMH_Cloneable Module Admin.lvclass">, "Accessors:External Launch"=w113:bool)  [unwired: 1 in, 1 out]
            n163 = case shown="True" w113 {
              tunnel: w114 -> [_ w125]
              tunnel: [_ w126] -> w117
              tunnel: w112 -> [w120 _]
              frame True {
                # "If externally launched, clicking the 'X' hides the panel, but doesn't close it."
                n164 = property on="Property Node" class="Mod Admin"(reference=w120) -> ("Accessors:Module ID"=w119:i32)  [unwired: 1 in, 2 out]
                n165 = call "Status Updated.vi"("Status"="Panel hidden." ("format string"), "Module ID"=w119) -> ("error out"=w118:errorcluster)  [unwired: 9 in]
                n166 = control-ref of="This VI"() -> (w122:refnum<vi>)
                n167 = call "Hide VI Panel.vi"("error in"=w118, "VI"=w122) -> ()  [unwired: 9 in, 1 out]
              }
              frame False {
                # "If run as a stand-alone VI, clicking the panel 'X' stops the VI."
                n168 = call-poly <vilib>:"Delacor_lib_QMH_Enqueue Message (poly).vi"("Priority Message? (F)"=TRUE, "Message"="Exit", "Message Queue in"=w125) -> ("error out"=w126:errorcluster)  [unwired: 7 in, 1 out]
              }
            }
            n169 = event-data ("Event Filter Node")("Discard?"=w116) -> ()  [unwired: 1 in, 1 out]
          }
          event User Event {
            # "Another Module called the \"select child\" API Method."
            n170 = event-data() -> ("Module ID"=w131:i32, "Hardware Selection"=w130:T6, "Wait Notifier"=w129:refnum<notifier>, "wait for reply"=w128:bool)  [unwired: 1 in]
            n171 = Bundle(cluster=T5 {"Module ID"=-1, "Hardware Selection"=enum."Wheatstone Bridge", "Wait Notifier"=refnum, "wait for reply"=FALSE} ("select child Argument"), "Module ID"=w131, "Hardware Selection"=w130, "Wait Notifier"=w129, "wait for reply"=w128) -> (w132:T5)
            n172 = call "Addressed to This Module.vi"("Module ID from Argument"=w131, "Module Admin"=w134) -> ("Addressed to this instance?"=w135:bool)  [unwired: 8 in, 1 out]
            n173 = case shown="True" w135 {
              tunnel: w136 -> [_ w140]
              tunnel: w132 -> [_ w138]
              tunnel: [_ w137] -> w127
              frame False {
              }
              frame True {
                n174 = call-poly <vilib>:"Delacor_lib_QMH_Enqueue Message (poly).vi"("Message Data"=w138, "Message"="select child", "Message Queue in"=w140) -> ("error out"=w137:errorcluster)  [unwired: 7 in, 1 out]
              }
            }
          }
          event User Event {
            # "Another Module called the \"read config\" API Method."
            n175 = event-data() -> ("Module ID"=w145:i32, "File Path"=w144:path, "Wait Notifier"=w143:refnum<notifier>, "wait for reply"=w142:bool)  [unwired: 1 in]
            n176 = Bundle(cluster=T7 {"Module ID"=-1, "File Path"=path "", "Wait Notifier"=refnum, "wait for reply"=FALSE} ("read config Argument"), "Module ID"=w145, "File Path"=w144, "Wait Notifier"=w143, "wait for reply"=w142) -> (w146:T7)
            n177 = call "Addressed to This Module.vi"("Module ID from Argument"=w145, "Module Admin"=w148) -> ("Addressed to this instance?"=w149:bool)  [unwired: 8 in, 1 out]
            n178 = case shown="True" w149 {
              tunnel: w150 -> [_ w154]
              tunnel: w146 -> [_ w152]
              tunnel: [_ w151] -> w141
              frame False {
              }
              frame True {
                n179 = call-poly <vilib>:"Delacor_lib_QMH_Enqueue Message (poly).vi"("Message Data"=w152, "Message"="read config", "Message Queue in"=w154) -> ("error out"=w151:errorcluster)  [unwired: 7 in, 1 out]
              }
            }
          }
          event User Event {
            # "Another Module called the \"init device\" API Method."
            n180 = event-data() -> ("Module ID"=w159:i32, "Variant"=w158:variant, "Wait Notifier"=w157:refnum<notifier>, "wait for reply"=w156:bool)  [unwired: 1 in]
            n181 = Bundle(cluster=T8 {"Module ID"=-1, "Variant"=variant, "Wait Notifier"=refnum, "wait for reply"=FALSE} ("init device Argument"), "Module ID"=w159, "Variant"=w158, "Wait Notifier"=w157, "wait for reply"=w156) -> (w160:T8)
            n182 = call "Addressed to This Module.vi"("Module ID from Argument"=w159, "Module Admin"=w162) -> ("Addressed to this instance?"=w163:bool)  [unwired: 8 in, 1 out]
            n183 = case shown="True" w163 {
              tunnel: w164 -> [_ w168]
              tunnel: w160 -> [_ w166]
              tunnel: [_ w165] -> w155
              frame False {
              }
              frame True {
                n184 = call-poly <vilib>:"Delacor_lib_QMH_Enqueue Message (poly).vi"("Message Data"=w166, "Message"="init device", "Message Queue in"=w168) -> ("error out"=w165:errorcluster)  [unwired: 7 in, 1 out]
              }
            }
          }
          event User Event {
            # "Another Module called the \"close\" API Method."
            n185 = event-data() -> ("Module ID"=w172:i32, "Wait Notifier"=w171:refnum<notifier>, "wait for reply"=w170:bool)  [unwired: 1 in]
            n186 = Bundle(cluster=T9 {"Module ID"=-1, "Wait Notifier"=refnum, "wait for reply"=FALSE} ("close Argument"), "Module ID"=w172, "Wait Notifier"=w171, "wait for reply"=w170) -> (w173:T9)
            n187 = call "Addressed to This Module.vi"("Module ID from Argument"=w172, "Module Admin"=w175) -> ("Addressed to this instance?"=w176:bool)  [unwired: 8 in, 1 out]
            n188 = case shown="True" w176 {
              tunnel: w177 -> [_ w181]
              tunnel: w173 -> [_ w179]
              tunnel: [_ w178] -> w169
              frame False {
              }
              frame True {
                n189 = call-poly <vilib>:"Delacor_lib_QMH_Enqueue Message (poly).vi"("Message Data"=w179, "Message"="close", "Message Queue in"=w181) -> ("error out"=w178:errorcluster)  [unwired: 7 in, 1 out]
              }
            }
          }
          event User Event {
            # "Another Module called the \"read data\" API Method."
            n190 = event-data() -> ("Module ID"=w185:i32, "Wait Notifier"=w184:refnum<notifier>, "wait for reply"=w183:bool)  [unwired: 1 in]
            n191 = Bundle(cluster=T10 {"Module ID"=-1, "Wait Notifier"=refnum, "wait for reply"=FALSE} ("read data Argument"), "Module ID"=w185, "Wait Notifier"=w184, "wait for reply"=w183) -> (w186:T10)
            n192 = call "Addressed to This Module.vi"("Module ID from Argument"=w185, "Module Admin"=w188) -> ("Addressed to this instance?"=w189:bool)  [unwired: 8 in, 1 out]
            n193 = case shown="True" w189 {
              tunnel: w190 -> [_ w194]
              tunnel: w186 -> [_ w192]
              tunnel: [_ w191] -> w182
              frame False {
              }
              frame True {
                n194 = call-poly <vilib>:"Delacor_lib_QMH_Enqueue Message (poly).vi"("Message Data"=w192, "Message"="read data", "Message Queue in"=w194) -> ("error out"=w191:errorcluster)  [unwired: 7 in, 1 out]
              }
            }
          }
          event User Event {
            # "Another Module called the \"read dvr\" API Method."
            n195 = event-data() -> ("Module ID"=w198:i32, "Wait Notifier"=w197:refnum<notifier>, "wait for reply"=w196:bool)  [unwired: 1 in]
            n196 = Bundle(cluster=T11 {"Module ID"=-1, "Wait Notifier"=refnum, "wait for reply"=FALSE} ("read dvr Argument"), "Module ID"=w198, "Wait Notifier"=w197, "wait for reply"=w196) -> (w199:T11)
            n197 = call "Addressed to This Module.vi"("Module ID from Argument"=w198, "Module Admin"=w201) -> ("Addressed to this instance?"=w202:bool)  [unwired: 8 in, 1 out]
            n198 = case shown="True" w202 {
              tunnel: w203 -> [_ w207]
              tunnel: w199 -> [_ w205]
              tunnel: [_ w204] -> w195
              frame False {
              }
              frame True {
                n199 = call-poly <vilib>:"Delacor_lib_QMH_Enqueue Message (poly).vi"("Message Data"=w205, "Message"="read dvr", "Message Queue in"=w207) -> ("error out"=w204:errorcluster)  [unwired: 7 in, 1 out]
              }
            }
          }
        }
        n200 = call-dynamic "Delacor_lib_QMH_Error Handler - Event Handling Loop.vi"("error in"=w42, "Message Queue in"=w36) -> ("dup error in"=w41:errorcluster)  [unwired: 8 in, 1 out]
      }
      n201 = while {
        tunnel: w19 -> [w31]
        stop <- w29 stop-if-true
        # "Data producing loop"
        n202 = control-ref of="Data Cluster"() -> (w34:refnum<vi>)
        n203 = property class="Clust (strict)"(reference=w34) -> ("Value"=w33:T1)  [unwired: 1 in, 2 out]
        n204 = property class="Mod Admin"(reference=w31) -> ("Accessors:Module ID"=w30:i32)  [unwired: 1 in, 2 out]
        n205 = Wait (ms)(milliseconds to wait=u32 1) -> ()  [unwired: 1 out]
        n206 = Unbundle By Name(w33) -> ("Status"=w32:string)
        n207 = case shown="\"Active\"" w32 {
          tunnel: w30 -> [_ w35]
          frame "inactive", Default {
          }
          frame "Active" {
            n208 = call "read data.vi"("Module ID"=w35) -> ()  [unwired: 9 in, 2 out]
          }
        }
        n209 = property on="Stop the VI" class="Bool (strict)"() -> ("Value"=w29:bool)  [unwired: 2 in, 2 out]
      }
    }
    frame Error {
      n210 = call "Synchronize Caller Events.vi"("Module Admin"=w442) -> ("Module Admin out"=w441:refnum<class "Delacor_lib_QMH_Cloneable Module Admin.lvclass">)  [unwired: 9 in, 1 out]
      n211 = property on="Property Node" class="Mod Admin"(reference=w441) -> ("Accessors:Module ID"=w440:i32)  [unwired: 1 in, 2 out]
      n212 = call-dynamic "Delacor_lib_QMH_Release Message Queue.vi"("error in"=w448, "Message Queue"=w439) -> ("error out"=w447:errorcluster)  [unwired: 9 in]
      n213 = call "Module Name--constant.vi"("Module ID"=w440) -> ("Module Name"=w445:string)  [unwired: 10 in]
      n214 = Format Into String(format string="An error occurred during initialization. %s is no longer running.", w445) -> (resulting string=w443:string)  [unwired: 2 in, 1 out]
      n215 = call "Error Reported.vi"("Additional Information"=w443, "Error"=w447, "Module ID"=w440) -> ()  [unwired: 8 in, 1 out]
    }
  }
  n216 = Merge Errors(w17, w16) -> (w18:errorcluster)
  n217 = call "Close Module.vi"("error in"=w18, "Wait for stop?"=w2, "Module Admin in"=w4) -> ("error out"=w14:errorcluster, "External Launch"=w1:bool, "Module Admin out"=w3:refnum<class "Delacor_lib_QMH_Cloneable Module Admin.lvclass">)  [unwired: 6 in]
  n218 = Unregister For Events(event registration refnum=w9, error in=w14) -> (error out=w13:errorcluster)
  "error out" <- w13
  n219 = case "External Launch?" shown="True" w1 {
    tunnel: w13 -> [_ w449]
    frame False {
    }
    frame True {
      n220 = case shown="No Error" w449 {
        frame No Error {
          n221 = invoke class="VI" method="FP.Close"() -> ()  [unwired: 3 in, 3 out]
        }
        frame Error {
          n222 = disable-structure shown="Default" {
            frame condition #0 (active) {
              n223 = invoke class="VI" method="FP.Open"("Activate"=TRUE ("Activate?")) -> ()  [unwired: 4 in, 5 out]
            }
            frame condition #1 {
              # "Don't show panel on error if running inside a built EXE."
            }
          }
        }
      }
    }
  }
  n224 = local write "Module Admin"(w3) -> ()
